vi "Convert from date-first Timestamp.vi"(4 "dttm string":string) -> (1 "Timestamp":timestamp)   [LabVIEW 2020, in "hse-db-ado.lvlib" / "ADO-DB-Driver.lvlib"]
doc: "Convert \"MM/DD/YYYY HH:MM:SS\" to timestamp\n\n____\nHAMPEL SOFTWARE ENGINEERING v1.4.0 (2023-12-19 09:52)"
uses:
  ADO-DB-Driver.lvlib
  <vilib>/Utility/miscctls.llb/LVDateTimeRec.ctl
panel:
  in  "?":T1
  # "Expects input string in the form \"MM/DD/YYYY HH:MM:SS\""
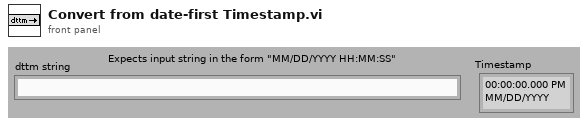
[diagram p1: front panel]
types:
  T1 = typedef "LVDateTimeRec.ctl" = cluster{"fractional second":dbl, "second":i32, "minute":i32, "hour":i32, "day of month":i32, "month":i32, "year":i32, "day of week":i32, "day of year":i32, "DST":i32}
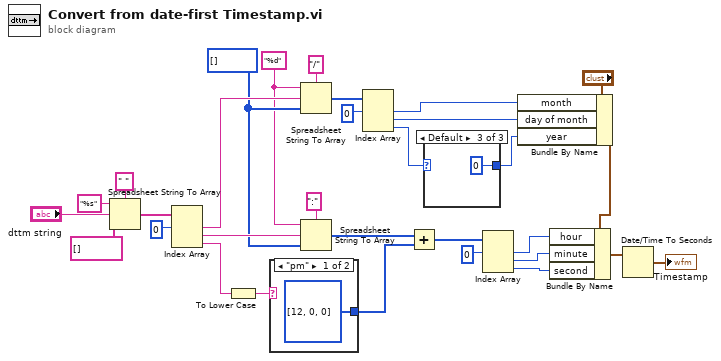
[diagram p0: block diagram]
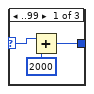
[diagram p2: hidden frame]
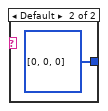
[diagram p4: hidden frame]
diagram:
  w20 = "%d" ("format string")
  w21 = i32[] [] ("array type (2D Dbl)")
  n1 = Spreadsheet String To Array(delimiter (Tab)=" ", format string="%s", spreadsheet string="dttm string", array type (2D Dbl)=string[] []) -> (array=w27:string[])
  n2 = Index Array(array=w27, index #1=0 ("index")) -> (element #1=w25:string, element #2=w22:string, element #3=w19:string)  [unwired: 2 in]
  n3 = To Lower Case(string=w19) -> (all lower case string=w18:string)
  n4 = case shown="\"pm\"" w18 {
    tunnel: [i32[] [12, 0, 0] ("array type (2D Dbl)") i32[] [0, 0, 0] ("array type (2D Dbl)")] -> w16
    frame "pm" {
    }
    frame Default {
    }
  }
  n5 = Spreadsheet String To Array(delimiter (Tab)="/", format string=w20, spreadsheet string=w25, array type (2D Dbl)=w21) -> (array=w14:i32[])
  n6 = Spreadsheet String To Array(delimiter (Tab)=":", format string=w20, spreadsheet string=w22, array type (2D Dbl)=w21) -> (array=w17:i32[])
  n7 = Index Array(array=w14, index #1=0 ("index")) -> (element #1=w11:i32, element #2=w10:i32, element #3=w4:i32)  [unwired: 2 in]
  n8 = Add(x=w17, y=w16) -> (x+y=w12:i32[])
  n9 = case shown="Default" w4 {
    selector: w4 -> [w34 w37 _]
    tunnel: [w36 w37 0 ("y")] -> w9
    frame ..99 {
      n10 = Add(x=w34, y=2000) -> (x+y=w36:i32)
    }
    frame 2000.. {
    }
    frame Default {
    }
  }
  n11 = Index Array(array=w12, index #1=0 ("index")) -> (element #1=w7:i32, element #2=w6:i32, element #3=w5:i32)  [unwired: 2 in]
  n12 = Bundle By Name(cluster="?", "month"=w11, "day of month"=w10, "year"=w9) -> (w8:T1)
  n13 = Bundle By Name(cluster=w8, "hour"=w7, "minute"=w6, "second"=w5) -> (w2:T1)
  n14 = Date/Time To Seconds(2:w2) -> (0:→"Timestamp":timestamp)  [unwired: 1 in]
